vi "Get hwnd.vi"(8 "Error in":errorcluster, 11 "LV MDI.lvclass":refnum<class "LV MDI.lvclass">) -> (0 "Error Out":errorcluster, 3 "LV MDI.lvclass  2":refnum<class "LV MDI.lvclass">)   [LabVIEW 2016, in "LV MDI.lvclass"]
uses:
  LV MDI.lvclass
  LV MDI.lvclass/LV MDI.ctl
  user32.dll
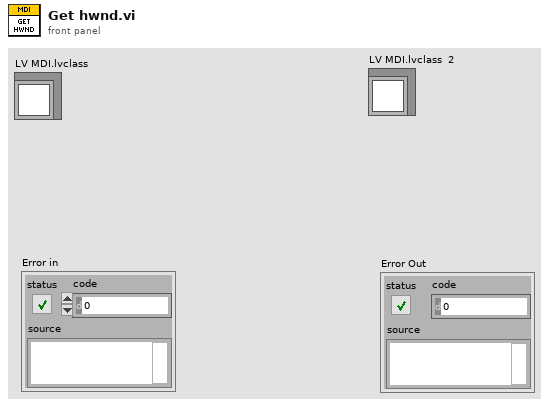
[diagram p1: front panel]
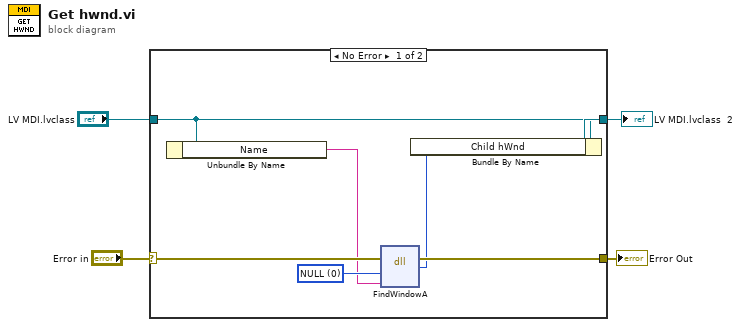
[diagram p0: block diagram]
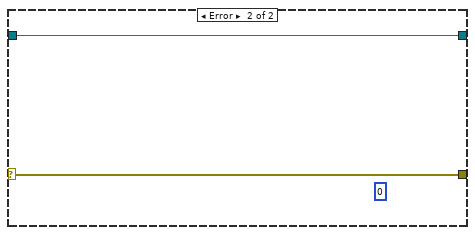
[diagram p2: hidden frame]
diagram:
  n1 = case shown="No Error" "Error in" {
    selector: "Error in" -> [w11 w13]
    tunnel: [w10 w13] -> w3
    tunnel: [w8 w12] -> w1
    tunnel: "LV MDI.lvclass" -> [w6 w12]
    frame No Error {
      w9 = 0 items=["NULL"]
      n2 = Unbundle By Name(w6) -> ("Name"=w5:string)
      n3 = dll-call lib="user32.dll" fn="FindWindowA"(error in=w11, "lpzsClassName"=w9, "lpzsWindowName"=w5) -> (error out=w10:errorcluster, "hwnd"=w7:u32)  [unwired: 4 in, 1 out]
      n4 = Bundle By Name(cluster=w6, "Child hWnd"=w7) -> (w8:refnum<class "LV MDI.lvclass">)
    }
    frame Error {
      (unwired) u32 0 ("hwnd")
    }
  }
  "Error Out" <- w3
  "LV MDI.lvclass  2" <- w1
